vi "Measure_Diode.vi"(8 "error in (no error)":errorcluster, 10 "Parameters":string, 11 "reference in":refnum<class "Test_Flux_Capacitor.lvclass">) -> (0 "error out":errorcluster, 2 "Result":dbl, 3 "reference out":refnum<class "Test_Flux_Capacitor.lvclass">)   [LabVIEW 2022 SP3, in "Test_Flux_Capacitor.lvlib" / "Test_Flux_Capacitor.lvclass"]
uses:
  Test_Flux_Capacitor.lvclass
  ParameterTypes/MeasureDiode.ctl
  ParameterTypes/PSU_SetV.vi
  ParameterTypes/DMM_DCV.vi
  <vilib>/Analysis/baseanly.llb/Mean (DBL).vi
  Components/SwitchBase.lvlibp/SwitchBase.lvclass
  Components/DMM_Keysight_34980A.lvlibp/DMM_Keysight_34980A.lvclass
  Components/PSU_Base.lvlibp/PSU_Base.lvclass
  <vilib>/Analysis/NI_AALBase.lvlib
  <vilib>/JDP Science/JSONtext/JSONtext.lvlib
panel:
  in  "Parameter_Type":T1={"Switch"="", "Wait (msec)"=0, "Scale"=0.0, "PSU"={"Chan"=0, "V"=0.0}, "DMM_DCV"={"Range "=enum."Auto", "Resolution"=enum."Default", "Samples"=1, "dt (s)"=0.0, "Timeout (s)"=10000.0}}
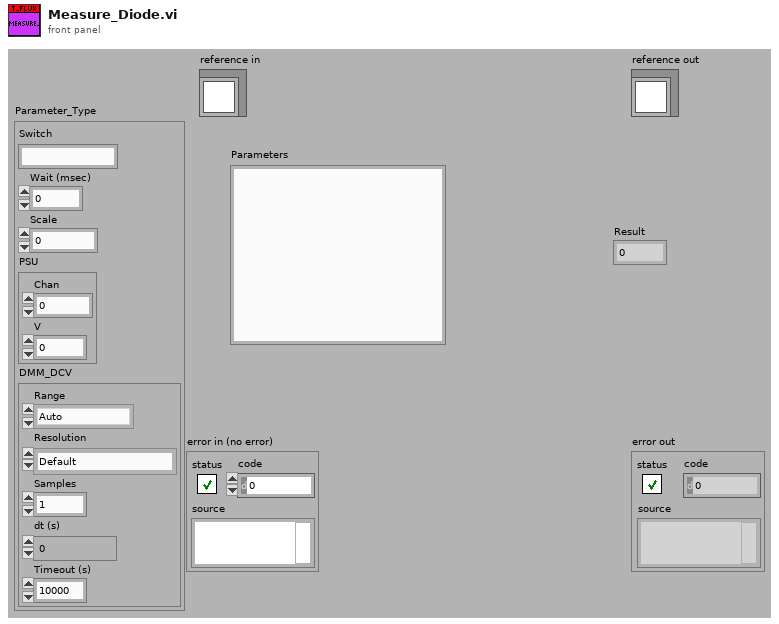
[diagram p1: front panel]
types:
  T1 = typedef "Test_Flux_Capacitor.lvlib/Test_Flux_Capacitor.lvclass/MeasureDiode.ctl" = cluster{"Switch":string, "Wait (msec)":u32, "Scale":dbl, "PSU":T2, "DMM_DCV":T3}
  T2 = typedef "Test_Flux_Capacitor.lvlib/Test_Flux_Capacitor.lvclass/PSU_SetV.vi" = cluster{"Chan":i32, "V":dbl}
  T3 = typedef "Test_Flux_Capacitor.lvlib/Test_Flux_Capacitor.lvclass/DMM_DCV.vi" = cluster{"Range ":enum16{"100 mV", "1 V", "10 V", "100 V", "300 V", "Auto", "Minimum", "Maximum"}, "Resolution":enum16{"4 1/2", "5 1/2", "6 1/2", "Least", "Highest", "Default"}, "Samples":u32, "dt (s)":dbl, "Timeout (s)":dbl}
  T4 = typedef "Test_Flux_Capacitor.lvlib/Test_Flux_Capacitor.lvclass/ObjectAttributes.ctl" = cluster{"Config":T5, "DMM":refnum<class "DMM_Keysight_34980A.lvclass">, "LCR":refnum<class "LCR_BK891.lvclass">, "PSU":refnum<class "PSU_Base.lvclass">, "Switch_Manager":refnum<class "SwitchBase.lvclass">, "FRAM":string, "Flux_Capacitor":refnum<class "Flux_Capacitor.lvclass">, "Frequency_Counter":refnum<class "Frequency_Counter_Base.lvclass">, "JTAG":refnum<class "JTAG_Base.lvclass">}
  T5 = typedef "Test_Flux_Capacitor.lvlib/Test_Flux_Capacitor.lvclass/Config.ctl" = cluster{"default":string}
  T6 = enum16{"100 mV", "1 V", "10 V", "100 V", "300 V", "Auto", "Minimum", "Maximum"}
  T7 = enum16{"4 1/2", "5 1/2", "6 1/2", "Least", "Highest", "Default"}
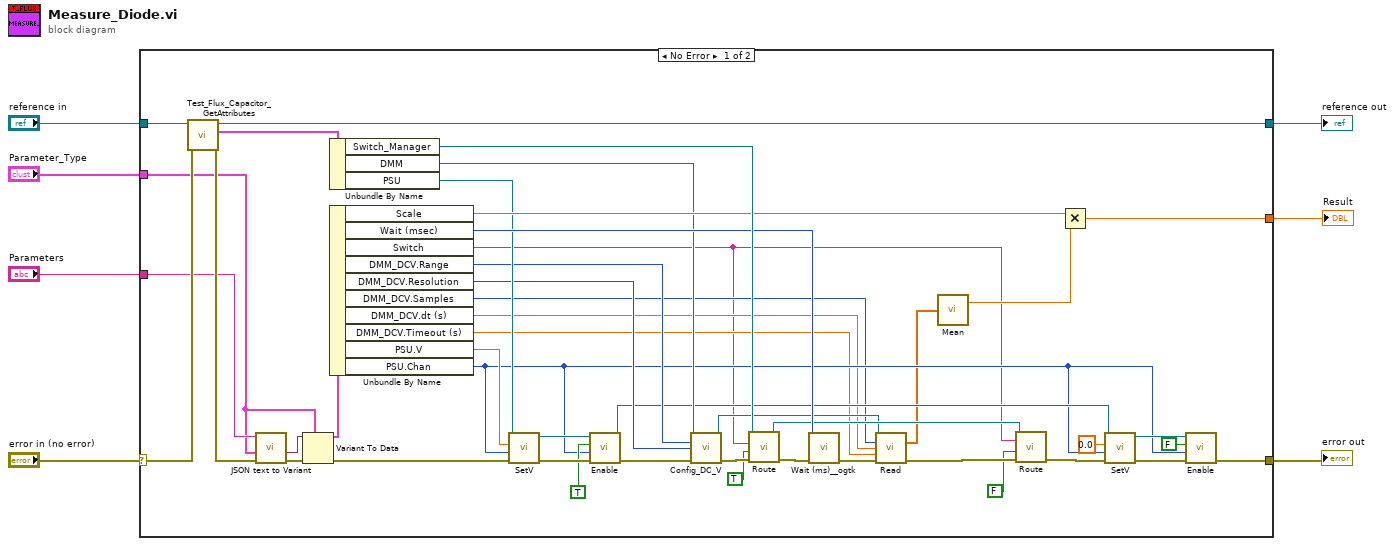
[diagram p0: block diagram]
diagram:
  n1 = case shown="No Error" "error in (no error)" {
    selector: "error in (no error)" -> [w53 w55]
    tunnel: [w24 w55] -> w6
    tunnel: [w51 w54] -> w4
    tunnel: "reference in" -> [w52 w54]
    tunnel: "Parameters" -> [w12 _]
    tunnel: "Parameter_Type" -> [w8 _]
    tunnel: [w43 _] -> w1
    frame No Error {
      n2 = call "Test_Flux_Capacitor_GetAttributes.vi"("error in (no error)"=w53, "reference in"=w52) -> ("error out"=w15:errorcluster, "Data"=w50:T4, "reference out"=w51:refnum<class "Test_Flux_Capacitor.lvclass">)  [unwired: 6 in, 1 out]
      n3 = call <vilib>:"JSON text to Variant.vi"("error in (no error)"=w15, "Data Type"=w8, "JSON"=w12) -> ("error out"=w14:errorcluster, "Variant out"=w13:variant)  [unwired: 7 in]
      n4 = Variant To Data(error in=w14, type=w8, Variant=w13) -> (data=w49:T1, error out=w33:errorcluster)
      n5 = Unbundle By Name(w50) -> ("Switch_Manager"=w48:refnum<class "SwitchBase.lvclass">, "DMM"=w37:refnum<class "DMM_Keysight_34980A.lvclass">, "PSU"=w40:refnum<class "PSU_Base.lvclass">)
      n6 = Unbundle By Name(w49) -> ("Scale"=w44:dbl, "Wait (msec)"=w46:u32, "Switch"=w11:string, "DMM_DCV.Range"=w39:T6, "DMM_DCV.Resolution"=w38:T7, "DMM_DCV.Samples"=w20:u32, "DMM_DCV.dt (s)"=w19:dbl, "DMM_DCV.Timeout (s)"=w18:dbl, "PSU.V"=w34:dbl, "PSU.Chan"=w21:i32)
      n7 = call-dynamic "SetV.vi"("error in (no error)"=w33, "Chan"=w21, "V"=w34, "reference in"=w40) -> ("error out"=w32:errorcluster, "reference in"=w30:refnum<class "PSU_Base.lvclass">)  [unwired: 6 in]
      n8 = call-dynamic "Enable.vi"("error in (no error)"=w32, "Chan"=w21, "Enable"=TRUE, "reference in"=w30) -> ("error out"=w31:errorcluster, "reference in"=w23:refnum<class "PSU_Base.lvclass">)  [unwired: 6 in]
      n9 = call-dynamic "Config_DC_V.vi"("reference in"=w37, "Range (5:Auto)"=w39, "Resolution (5:Default)"=w38, "error in (no error)"=w31) -> ("reference in"=w35:refnum<class "DMM_Keysight_34980A.lvclass">, "error out"=w36:errorcluster)  [unwired: 10 in]
      n10 = call-dynamic "Route.vi"("error in (no error)"=w36, "Connect"=TRUE, "channel 1"=w11, "reference in"=w48) -> ("error out"=w47:errorcluster, "reference in"=w45:refnum<class "SwitchBase.lvclass">)  [unwired: 6 in]
      n11 = call <userlib>:"Wait (ms)__ogtk.vi"("error in (no error)"=w47, "milliseconds to wait"=w46) -> ("error out"=w42:errorcluster)  [unwired: 8 in, 1 out]
      n12 = call-dynamic "Read.vi"("reference in"=w35, "Samples"=w20, "dt"=w19, "Timeout (10 s)"=w18, "error in (no error)"=w42) -> ("Measurement"=w17:dbl[], "error out"=w41:errorcluster)  [unwired: 7 in, 2 out]
      n13 = call-poly <vilib>:"Mean.vi"("X"=w17) -> ("mean"=w16:dbl)  [unwired: 1 out]
      n14 = call-dynamic "Route.vi"("error in (no error)"=w41, "Connect"=FALSE ("Enable"), "channel 1"=w11, "reference in"=w45) -> ("error out"=w25:errorcluster)  [unwired: 6 in, 1 out]
      n15 = Multiply(x=w44, y=w16) -> (x*y=w43:dbl)
      n16 = call-dynamic "SetV.vi"("error in (no error)"=w25, "Chan"=w21, "V"=0.0, "reference in"=w23) -> ("error out"=w28:errorcluster, "reference in"=w27:refnum<class "PSU_Base.lvclass">)  [unwired: 6 in]
      n17 = call-dynamic "Enable.vi"("error in (no error)"=w28, "Chan"=w21, "Enable"=FALSE, "reference in"=w27) -> ("error out"=w24:errorcluster)  [unwired: 6 in, 1 out]
    }
    frame Error {
    }
  }
  "Result" <- w1
  "error out" <- w6
  "reference out" <- w4
